vi "Create Message-Enqueuer References.vi"(8 "error in (no error)":errorcluster) -> (0 "error out":errorcluster, 3 "API":T1)   [LabVIEW 2018, in "Actor.lvclass"]
uses:
  Actor.lvclass
  Message-Enqueuer References.ctl
  Stop.ctl
  Launch.ctl
  Did Initialize.ctl
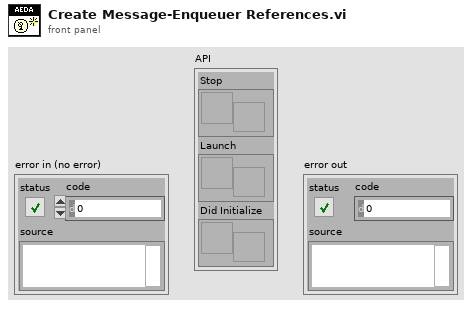
[diagram p1: front panel]
types:
  T1 = typedef "Actor.lvclass/Message-Enqueuer References.ctl" = cluster{"Stop":refnum<user-event>, "Launch":refnum<user-event>, "Did Initialize":refnum<user-event>}
  T2 = typedef "Actor.lvclass/Launch.ctl" = cluster{"Caller":refnum<vi>}
  T3 = typedef "Actor.lvclass/Did Initialize.ctl" = cluster{"State":refnum<class "Actor.lvclass">}
  T4 = typedef "Actor.lvclass/Stop.ctl" = cluster{"Type":enum16{"Normal", "Emergency"}}
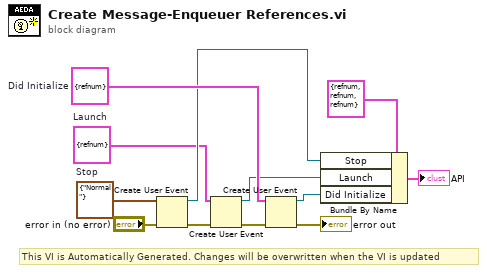
[diagram p0: block diagram]
diagram:
  w1 = T2 {"Caller"=refnum}  # Launch
  w12 = T3 {"State"=refnum}  # Did Initialize
  w11 = T4 {"Type"=enum."Normal"}  # Stop
  # "This VI is Automatically Generated. Changes will be overwritten when the VI is updated"
  n1 = Create User Event(user event datatype=w11, error in="error in (no error)") -> (user event=w8:refnum<user-event>, error out=w5:errorcluster)
  n2 = Create User Event(user event datatype=w1, error in=w5) -> (user event=w2:refnum<user-event>, error out=w4:errorcluster)
  n3 = Create User Event(user event datatype=w12, error in=w4) -> (user event=w6:refnum<user-event>, error out=→"error out":errorcluster)
  n4 = Bundle By Name(cluster=T1 {"Stop"=refnum, "Launch"=refnum, "Did Initialize"=refnum} ("Actor-Events"), "Stop"=w8, "Launch"=w2, "Did Initialize"=w6) -> (→"API":T1)
